vi "Part 2.vi"(11 "Input":string) -> (3 "Output":i64)   [LabVIEW 2021]
uses:
  <userlib>/_OpenG.lib/string/string.llb/Convert EOLs (String)__ogtk.vi
panel:
  out "Count":i32
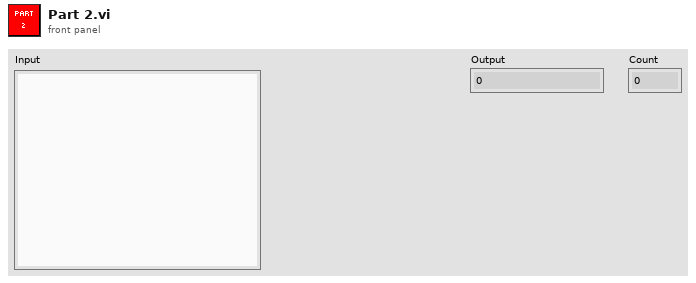
[diagram p1: front panel]
types:
  T1 = map{cluster{"Config":u8[], "Numbers":i64[]}, i64}
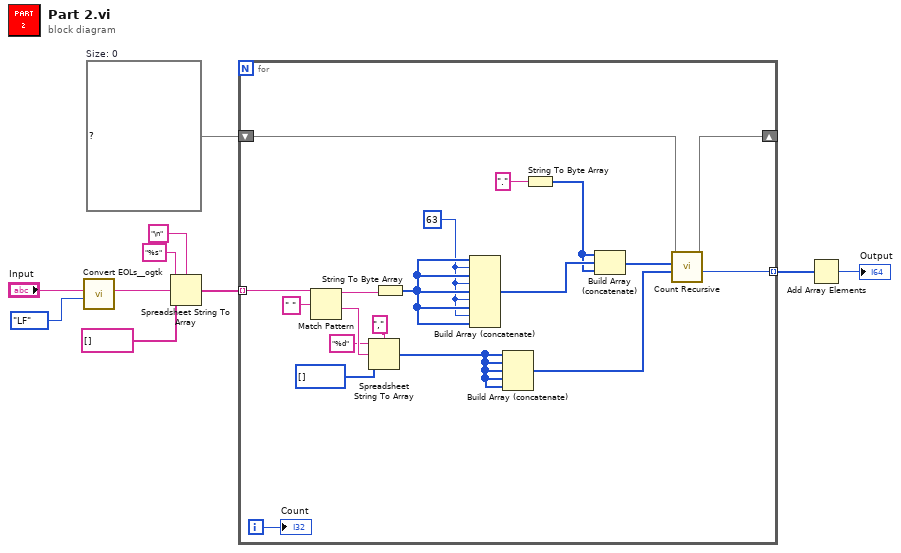
[diagram p0: block diagram]
diagram:
  w1 = T1 {}  # Size: 0
  n1 = call-poly <userlib>:"Convert EOLs__ogtk.vi"("Convert to:"=enum16{"CR", "LF", "CRLF"}."LF", "String in"="Input") -> ("String out"=w6:string)  [unwired: 9 in]
  n2 = Spreadsheet String To Array(delimiter (Tab)="\n", format string="%s", spreadsheet string=w6, array type (2D Dbl)=string[] []) -> (array=w4:string[])
  n3 = for {
    tunnel: w4 -> [w29] mode=indexing
    tunnel: [w15] -> w3 mode=indexing
    shift-right: [w16] -> _
    shift-left: w1 -> [w18]
    i -> [w22]
    w13 = u8 63 ("Element Data")
    n4 = Match Pattern(string=w29, regular expression=" ") -> (before substring=w23:string, after substring=w27:string)  [unwired: 1 in, 2 out]
    n5 = Spreadsheet String To Array(delimiter (Tab)=",", format string="%d", spreadsheet string=w27, array type (2D Dbl)=i64[] []) -> (array=w11:i64[])
    n6 = String To Byte Array(string=w23) -> (unsigned byte array=w14:u8[])
    n7 = Build Array (concatenate)(w14, w13, w14, w13, w14, w13, w14, w13, w14) -> (w21:u8[])
    n8 = Build Array (concatenate)(w11, w11, w11, w11, w11) -> (w12:i64[])
    n9 = String To Byte Array(string=".") -> (unsigned byte array=w19:u8[])
    n10 = Build Array (concatenate)(w19, w21, w19) -> (w17:u8[])
    n11 = call "Count Recursive.vi"("Numbers"=w12, "Config"=w17, "Map In"=w18) -> ("Count"=w15:i64, "Map Out"=w16:T1)  [unwired: 7 in]
    "Count" <- w22
  }
  n12 = Add Array Elements(numeric array=w3) -> (sum=→"Output":i64)
